vi "Check Dist to Starting WP.vi"   [LabVIEW 2009]
uses:
  <vilib>/Platform/TimedLoop/XDataNode/XDataNode.xnode
  <vilib>/Platform/TimedLoop/XDataNode/loadlvalarms.vi
  <vilib>/Platform/TimedLoop/XDataNode/timing_clust.ctl
  <vilib>/Platform/TimedLoop/XDataNode/nitl_modes.ctl
  <vilib>/Platform/TimedLoop/XDataNode/wakeup.ctl
  Functional Global Variables/Actions for FG's.ctl
  <vilib>/Platform/TimedLoop/XDataNode/XDNodeRunTimeDep.lvlib
types:
  T1 = typedef "XDNodeRunTimeDep.lvlib/timing_clust.ctl" = cluster{"Expected End [f-1]":u64, "Actual End [f-1]":u64, "Finished Late? [f-1]":bool, "Expected End [i-1]":u64, "Actual End [i-1]":u64, "Finished Late? [i-1]":bool, "Expected Start [i]":u64, "Actual Start [i]":u64, "Expected Start [f]":u64, "Actual Start [f]":u64, "Source Name":string, "Structure Name":string, "Period":i64, "Deadline":i64, "Offset":i64, "Start":i64, "Priority":i32, "Timeout":i32, "Mode":T2, "Wakeup Reason":T3, "Error":errorcluster, "Source Type":string, "Secondary Source Type":string, "Global End Time":u64, "Global Start Time":u64, "Frame Duration":u64, "Iteration Duration":u64, "Assigned CPU":i32, "I/O Scan Engine Mode":u32}
  T2 = typedef "XDNodeRunTimeDep.lvlib/nitl_modes.ctl" = enum32{"No Change", "Process missed periods, maintain original phase", "Discard missed periods, maintain original phase", "Process missed periods, ignore original phase", "Discard missed periods, ignore original phase"}
  T3 = typedef "XDNodeRunTimeDep.lvlib/wakeup.ctl" = enum32{"Normal", "Aborted", "Asynchronous wakeup", "Timing source error", "Timed loop error", "Timeout"}
  T4 = typedef "Actions for FG's.ctl" = enum16{"Read", "Write"}
  T5 = typedef "GPS Data.ctl" = cluster{"Latitude":dbl, "Longitude":dbl}
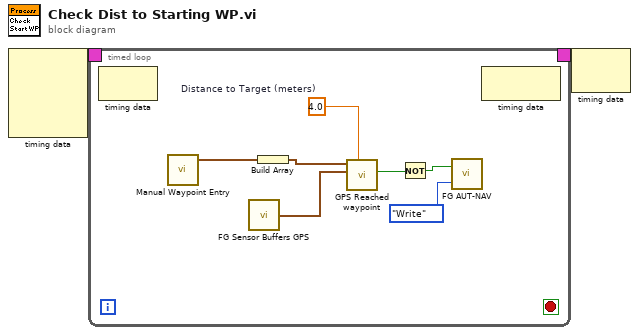
[diagram p0: block diagram]
diagram:
  n1 = node-c288() -> (w2:T1)  [unwired: 4 in]
  n2 = timed-loop {
    timing: w2 -> [_]
    timing-out: [_] -> w1
    stop <- _ stop-if-true
    w6 = 4.0  # Distance to Target (meters)
    n3 = node-c288() -> ()  [unwired: 1 in, 1 out]
    n4 = call "Manual Waypoint Entry.vi"() -> ("Nav Course Start Location"=w9:T5)  [unwired: 3 in, 2 out]
    n5 = call "FG Sensor Buffers GPS.vi"() -> ("GPS Buffer out"=w7:T5)  [unwired: 2 in]
    n6 = Build Array(w9) -> (w8:T5[])
    n7 = call "GPS Reached waypoint.vi"("Required distance to target (meters)"=w6, "Current Co-ordinates"=w7, "Waypoint List In"=w8) -> ("Reached waypoint?"=w5:bool)  [unwired: 5 in, 3 out]
    n8 = Not(x=w5) -> (.not. x?=w4:bool)
    n9 = call "FG AUT-NAV.vi"("FG Action (Read)"=Actions_for_FG's."Write", "Aut/!Nav in"=w4) -> ()  [unwired: 1 out]
    n10 = node-c288() -> ()  [unwired: 1 in, 1 out]
  }
  n11 = node-c288(w1) -> ()  [unwired: 1 out]
